vi "Init.vi"(3 "Container State":T6={"Indicator?"=TRUE, "Run Mode?"=FALSE, " Refnum"=refnum}, 4 "Previous State":variant=variant(cluster{"Draw Options":cluster{"Background Color":u32, "Grid Color":u32, "Angle Units":enum16{"Radians", "Degrees"}, "Draw Solid Background":bool, "Draw Grid":bool, "Grid Spacing":dbl, "AutoScale":bool, "Fit to Radius":dbl, "data row options":cluster{"point color":u32, "line color":u32, "draw points":bool, "draw lines":bool, "point pixel size":u16, "max line distance":dbl, "line pixel width":u16}[]}} {"Draw Options"={"Background Color"=16777215, "Grid Color"=13816530, "Angle Units"=enum."Degrees", "Draw Solid Background"=TRUE, "Draw Grid"=TRUE, "Grid Spacing"=1.0, "AutoScale"=TRUE, "Fit to Radius"=1.0, "data row options"=[{"point color"=16711680, "line color"=16711680, "draw points"=TRUE, "draw lines"=TRUE, "point pixel size"=5, "max line distance"=inf, "line pixel width"=2}, {"point color"=1985280, "line color"=1985280, "draw points"=TRUE, "draw lines"=TRUE, "point pixel size"=5, "max line distance"=1.0, "line pixel width"=2}]}}), 5 "Previous Version":T5={"Major"=1, "Minor"=0, "Fix"=0, "Build"=0}) -> (2 "Current State":T1={"Draw Options"={"Background Color"=16777215, "Grid Color"=13816530, "Angle Units"=enum."Degrees", "Draw Solid Background"=TRUE, "Draw Grid"=TRUE, "Grid Spacing"=1.0, "AutoScale"=TRUE, "Fit to Radius"=1.0, "data row options"=[{"point color"=16711680, "line color"=16711680, "draw points"=TRUE, "draw lines"=TRUE, "point pixel size"=5, "max line distance"=inf, "line pixel width"=2}, {"point color"=1985280, "line color"=1985280, "draw points"=TRUE, "draw lines"=TRUE, "point pixel size"=5, "max line distance"=1.0, "line pixel width"=2}]}})   [LabVIEW 2017, in "NI_Robotics_2D Rangefinder.xctl"]
uses:
  <vilib>/robotics/Controls/2D Rangefinder/NI_Robotics_2D Rangefinder.xctl
  <vilib>/robotics/Controls/2D Rangefinder/_2D Rangefinder Support Files/State.ctl
  <vilib>/robotics/Controls/2D Rangefinder/2D Rangefinder Picture/Draw Options.ctl
  <vilib>/robotics/Controls/Utilities/Angle Units.ctl
  <vilib>/robotics/Controls/2D Rangefinder/2D Rangefinder Picture/Data Row Options.ctl
  <vilib>/_xctls/Container State.ctl
  <vilib>/_xctls/Version.ctl
  <vilib>/robotics/Controls/2D Rangefinder/2D Rangefinder Picture/NI_Robotics_2D Rangefinder Picture.lvlib
  <vilib>/_xctls/XControlSupport.lvlib
  <vilib>/robotics/Controls/Utilities/NI_Robotics_Control Utilities.lvlib
panel:
  in  "Default Indicator State":T1={"Draw Options"={"Background Color"=16777215, "Grid Color"=13816530, "Angle Units"=enum."Degrees", "Draw Solid Background"=TRUE, "Draw Grid"=TRUE, "Grid Spacing"=0.25, "AutoScale"=FALSE, "Fit to Radius"=1.0, "data row options"=[]}}
  in  "Default Control State":T1={"Draw Options"={"Background Color"=16777215, "Grid Color"=13816530, "Angle Units"=enum."Degrees", "Draw Solid Background"=TRUE, "Draw Grid"=TRUE, "Grid Spacing"=0.25, "AutoScale"=FALSE, "Fit to Radius"=1.0, "data row options"=[]}}
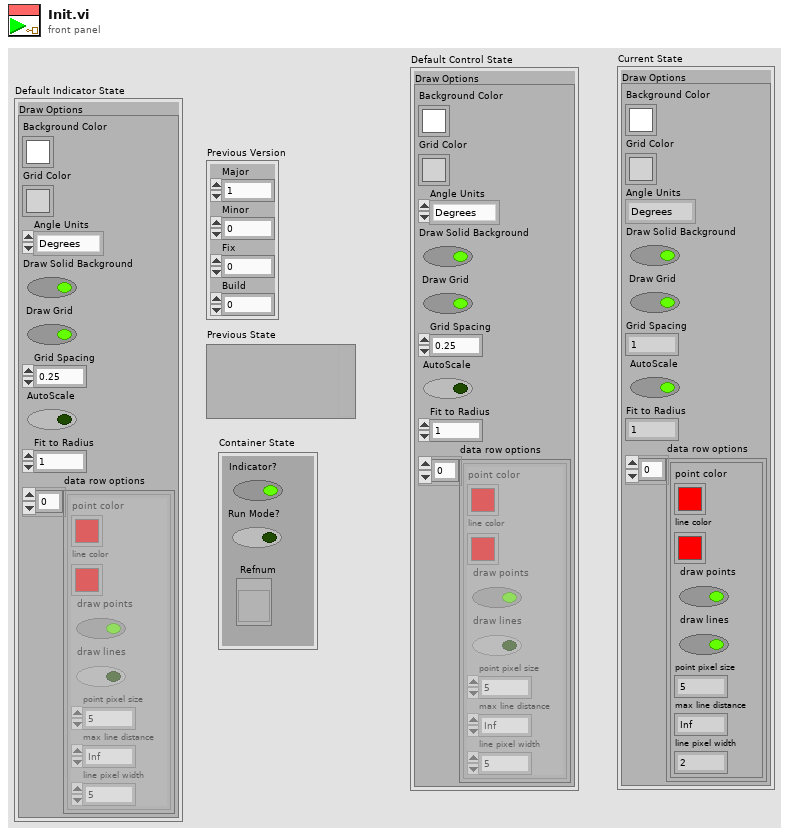
[diagram p1: front panel]
types:
  T1 = typedef "NI_Robotics_2D Rangefinder.xctl/State.ctl" = cluster{"Draw Options":T2}
  T2 = typedef "NI_Robotics_2D Rangefinder Picture.lvlib/Draw Options.ctl" = cluster{"Background Color":u32, "Grid Color":u32, "Angle Units":T3, "Draw Solid Background":bool, "Draw Grid":bool, "Grid Spacing":dbl, "AutoScale":bool, "Fit to Radius":dbl, "data row options":T4[]}
  T3 = typedef "NI_Robotics_Control Utilities.lvlib/Angle Units.ctl" = enum16{"Radians", "Degrees"}
  T4 = typedef "NI_Robotics_2D Rangefinder Picture.lvlib/Data Row Options.ctl" = cluster{"point color":u32, "line color":u32, "draw points":bool, "draw lines":bool, "point pixel size":u16, "max line distance":dbl, "line pixel width":u16}
  T5 = typedef "XControlSupport.lvlib/Version.ctl" = cluster{"Major":u16, "Minor":u16, "Fix":u16, "Build":u16}
  T6 = typedef "XControlSupport.lvlib/Container State.ctl" = cluster{"Indicator?":bool, "Run Mode?":bool, " Refnum":refnum<vi>}
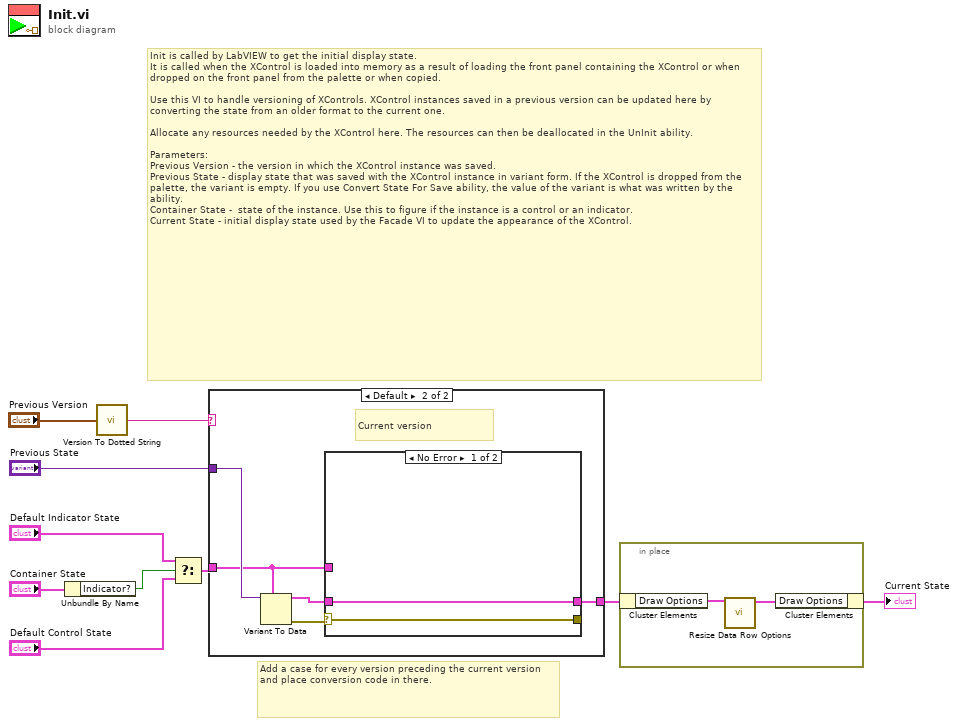
[diagram p0: block diagram]
diagram:
  # "Add a case for every version preceding the current version and place conversion code in there."
  # "Init is called by LabVIEW to get the initial display state.\nIt is called when the XControl is loaded into memory as a result of loading the front panel containing the XControl or when dropped on the front panel from the palette or when copied.\n\nUse this VI to handle versioning of XControls. XControl instances saved in a previous version can be updated here by converting the state from an older format to the current one.\n\nAllocate any resources needed by the XControl here. The resources can then be deallocated in the UnInit ability.\n\nParameters:\nPrevious Version - the version in which the XControl instance was saved.\nPrevious State - display state that was saved with the XControl instance in variant form. If the XControl is dropped from the palette, the variant is empty. If you use Convert State For Save ability, the value of the variant is what was written by the ability. \nContainer State -  state of the instance. Use this to figure if the instance is a control or an indicator.\nCurrent State - initial display state used by the Facade VI to update the appearance of the XControl."
  n1 = Unbundle By Name("Container State") -> ("Indicator?"=w6:bool)
  n2 = call <vilib>:"Version To Dotted String.vi"("Version"="Previous Version") -> ("String Version"=w3:string)
  n3 = Select(t="Default Indicator State", s=w6, f="Default Control State") -> (s? t:f=w5:T1)
  n4 = case shown="Default" w3 {
    tunnel: "Previous State" -> [_ w16]
    tunnel: [w11 w12] -> w2
    tunnel: w5 -> [w11 w13]
    frame "0.0.0.0" {
      # "Just created, use default state"
    }
    frame Default {
      # "Current version"
      n5 = Variant To Data(type=w13, Variant=w16) -> (data=w14:T1, error out=w15:errorcluster)  [unwired: 1 in]
      n6 = case shown="No Error" w15 {
        selector: w15 -> [w18 w19]
        tunnel: w14 -> [w17 _]
        tunnel: [w17 w20] -> w12
        tunnel: w13 -> [_ w20]
        tunnel: [w18 w19] -> _
        frame No Error {
        }
        frame Error {
          # "Error converting previously \nsaved state. Use default instead."
        }
      }
    }
  }
  n7 = in-place {
    n8 = in-place-cluster #1(w2) -> ("Draw Options"=w22:T2)
    n9 = call <vilib>:"Resize Data Row Options.vi"("draw options in"=w22) -> ("draw options out"=w21:T2)  [unwired: 10 in]
    n10 = in-place-cluster #1("Draw Options"=w21) -> (→"Current State":T1)
  }
